vi "Kinect Track Demo.vi"() -> ()   [LabVIEW 2010]
uses:
  Kinect_API.lvlib
  labview-trunk/vi/clearpath_interface.lvlib
  <vilib>/Platform/TimedLoop/XDataNode/wakeup.ctl
  <vilib>/Platform/TimedLoop/XDataNode/XDNodeRunTimeDep.lvlib
  <vilib>/Platform/TimedLoop/XDataNode/nitl_modes.ctl
  <vilib>/Platform/TimedLoop/XDataNode/timing_clust.ctl
  <vilib>/Platform/TimedLoop/XDataNode/XDataNode.xnode
  cpp_lv.dll
panel:
  in  "Stop Husky":bool=TRUE
  in  "Tab Control":T1(tab)
  out "Depth":T2(plugin-control)
  out "Video":T2(plugin-control)
  in  "Wait For Next Image?":bool
  out "Depth Image Pixels (U16)":u16[][](array[numeric])
  out "Video Image Pixels (U32)":u32[][](array[numeric])
  out "Image Is New? (Video)":bool
  out "Image Is New? (Depth)":bool
  in  "Remove Zeros?":bool=TRUE
  in  "Focal Length in Pixels":dbl=285.63
  out "Iteration Delay":u32
  out "Mean Delay (N=100)":dbl
  out "Approx. FPS":dbl
  in  "Wall Buffer":dbl=0.7 min=0.0 step=0.1
  in  "FollowModeOn":bool=TRUE
  out "Linear Velocity":dbl(knob) scale=-1.0..1.0
  out "Angular Velocity":dbl(knob) scale=2.0..-2.0
  in  "Serial Port":refnum<visa-resource-name>="COM1"
  in  "Linear Speed":dbl=0.3 min=0.0 max=1.0 step=0.1
  in  "Angular Speed":dbl=0.2 min=0.0 max=2.0 step=0.1
  in  "Window Size":dbl=0.5 min=0.0 step=0.1
  in  "stop":bool
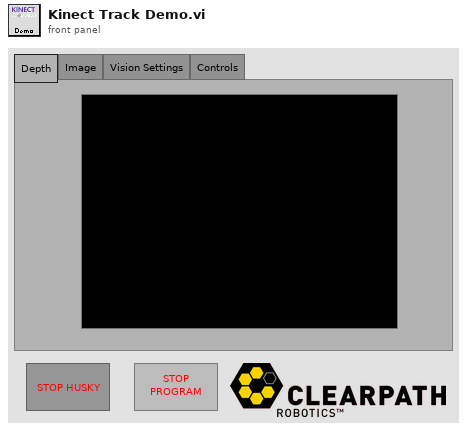
[diagram p1: front panel]
types:
  T1 = enum32{"Depth", "Image", "Vision Settings", "Controls"}
  T2 = typedef "IMAQ Image.ctl" = refnum<image>
  T3 = cluster{"Xmit Queue":refnum<queue>, "Data Queue":refnum<queue>, "VISA resource name out":refnum<visa-resource-name>, "error out":errorcluster, "Message Data Cluster":cluster{"\nChar Idx":u8, "Num. Char Rem":u8, "Write Index":u8, "Read Index":u8, "Message Data Buffer":u8[][]}}
  T4 = typedef "XDNodeRunTimeDep.lvlib/timing_clust.ctl" = cluster{"Expected End [f-1]":u64, "Actual End [f-1]":u64, "Finished Late? [f-1]":bool, "Expected End [i-1]":u64, "Actual End [i-1]":u64, "Finished Late? [i-1]":bool, "Expected Start [i]":u64, "Actual Start [i]":u64, "Expected Start [f]":u64, "Actual Start [f]":u64, "Source Name":string, "Structure Name":string, "Period":i64, "Deadline":i64, "Offset":i64, "Start":i64, "Priority":i32, "Timeout":i32, "Mode":T5, "Wakeup Reason":T6, "Error":errorcluster, "Source Type":string, "Secondary Source Type":string, "Global End Time":u64, "Global Start Time":u64, "Frame Duration":u64, "Iteration Duration":u64, "Assigned CPU":i32, "I/O Scan Engine Mode":u32}
  T5 = typedef "XDNodeRunTimeDep.lvlib/nitl_modes.ctl" = enum32{"No Change", "Process missed periods, maintain original phase", "Discard missed periods, maintain original phase", "Process missed periods, ignore original phase", "Discard missed periods, ignore original phase"}
  T6 = typedef "XDNodeRunTimeDep.lvlib/wakeup.ctl" = enum32{"Normal", "Aborted", "Asynchronous wakeup", "Timing source error", "Timed loop error", "Timeout"}
  T7 = cluster{"queue out":refnum<queue>, "queue out":refnum<queue>}
  T8 = cluster{"new reference":refnum<k24>, "DepthStream":refnum<k24>, "VideoStream":refnum<k24>, "Event Callback":refnum<k27>, "Event Callback":refnum<k27>}
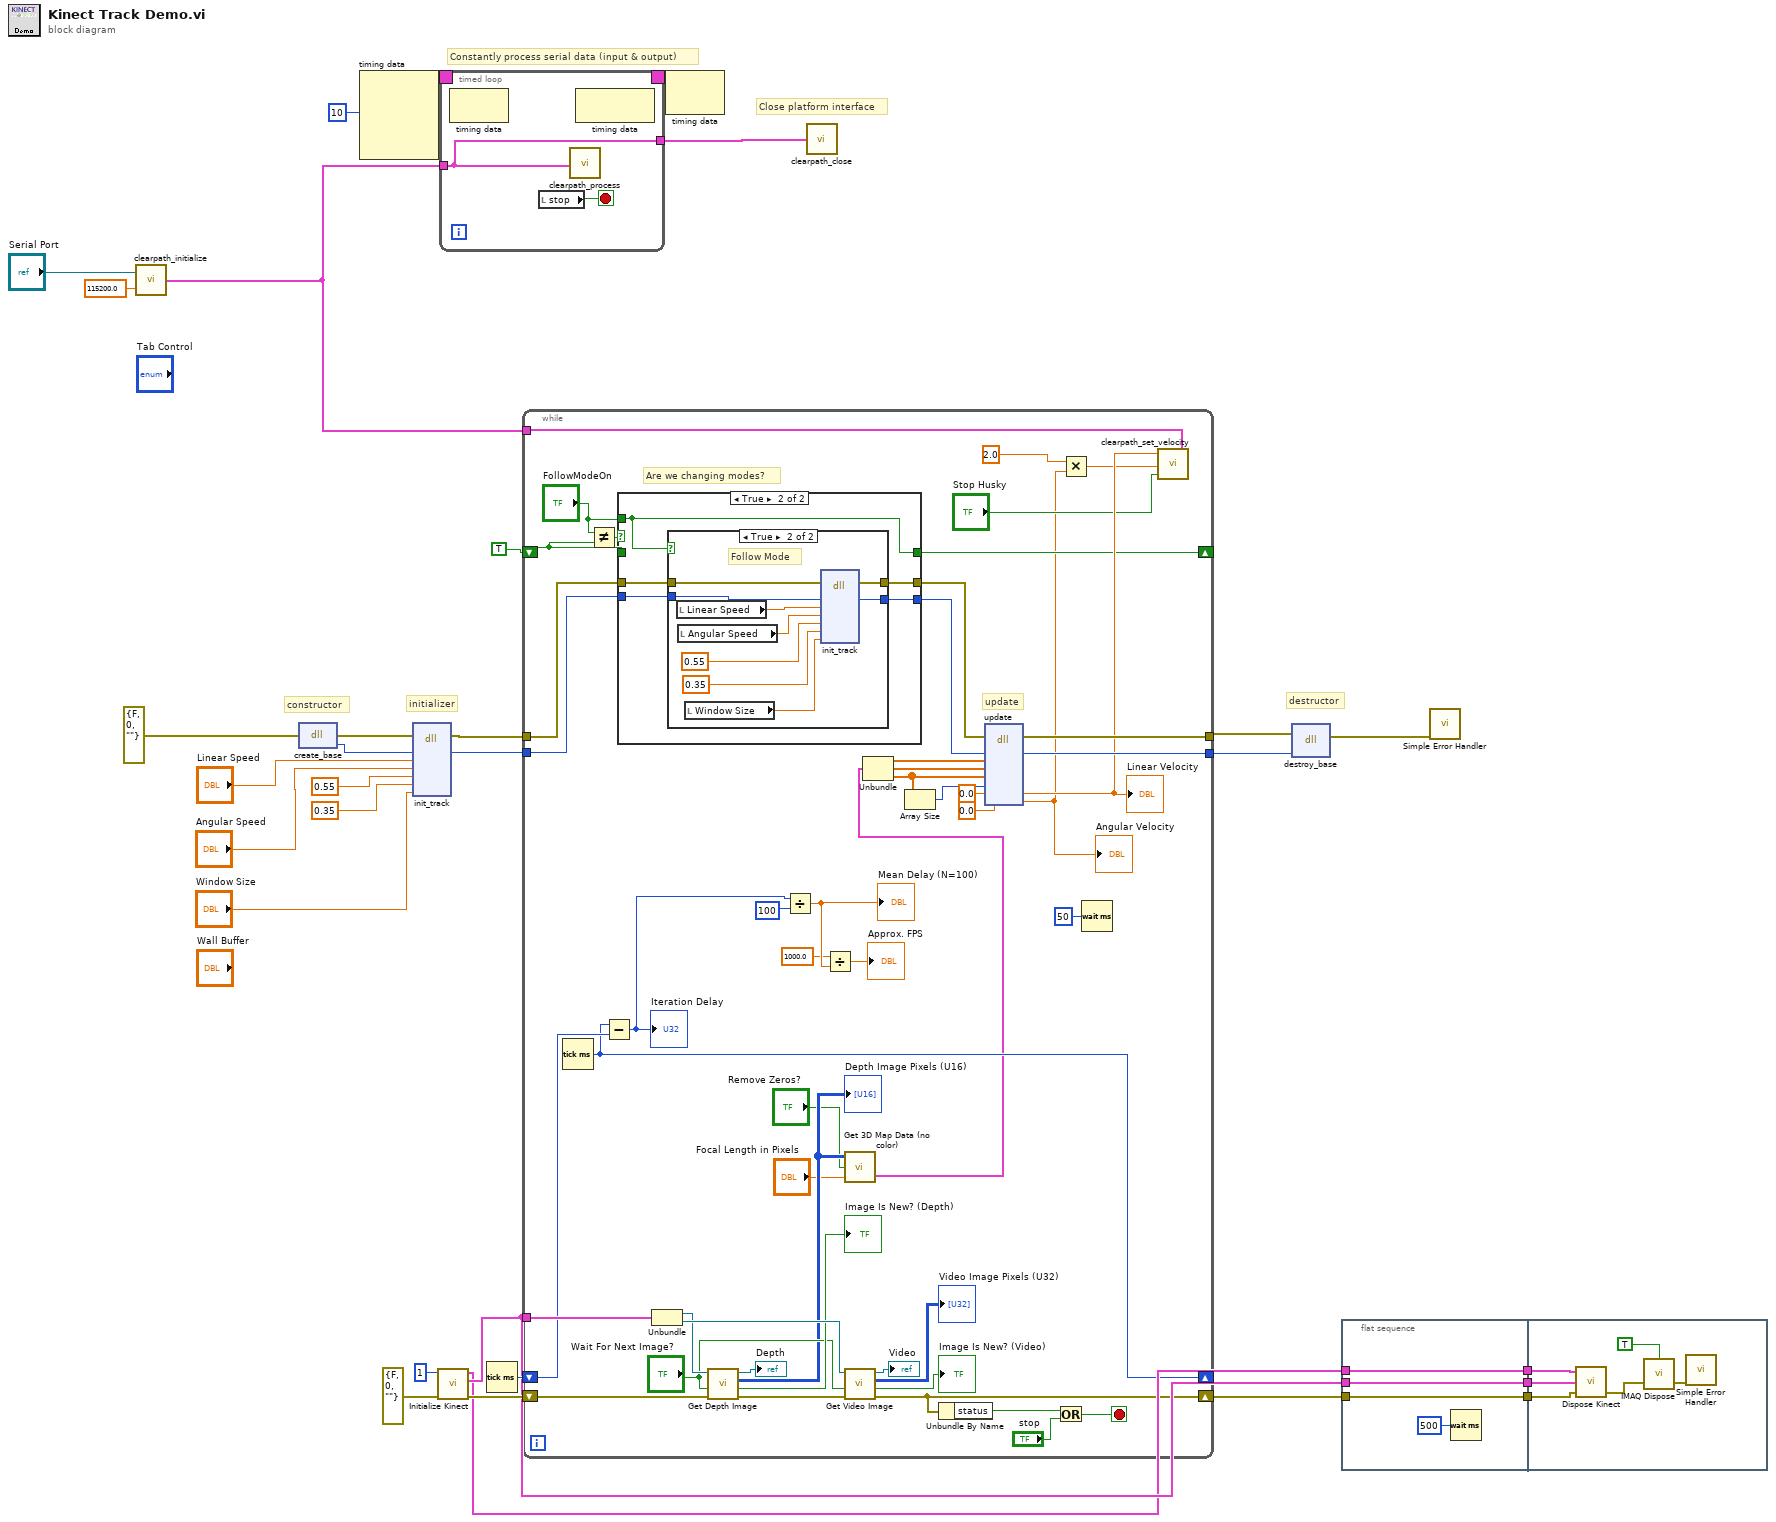
[diagram p0: block diagram]
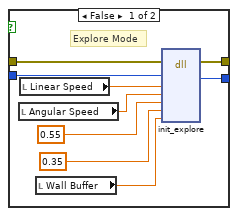
[diagram p3: hidden frame]
diagram:
  # "destructor"
  # "initializer"
  # "constructor"
  # "Constantly process serial data (input & output)"
  # "Close platform interface"
  n1 = call "clearpath_initialize.vi"("Baud rate"=115200.0, "VISA resource name"="Serial Port") -> ("ClearpathComm"=w31:T3)
  n2 = dll-call lib="C:/Users/clearpath/Desktop/Kinect Demo/cpp_lv.dll" fn="create_base"(error in=errorcluster {"status"=FALSE, "code"=0, "source"=""} ("error in (no error)")) -> (error out=w9:errorcluster, "LV_ref"=w8:u32)  [unwired: 2 in, 1 out]
  n3 = node-c288(i64 10 ("Period")) -> (w15:T4)  [unwired: 3 in]
  n4 = dll-call lib="C:/Users/clearpath/Desktop/Kinect Demo/cpp_lv.dll" fn="init_track"(error in=w9, "LV_ref"=w8, "lin_speed"="Linear Speed", "ang_speed"="Angular Speed", "cam_height"=0.55, "cam_z_trans"=0.35, "window_size"="Window Size") -> (error out=w18:errorcluster, "LV_ref"=w17:u32)  [unwired: 8 in, 1 out]
  n5 = call "Initialize Kinect.vi"("error in (no error)"=errorcluster {"status"=FALSE, "code"=0, "source"=""}, "Buffer Size"=1) -> ("error out"=w27:errorcluster, "Queues Out"=w23:T7, "References"=w22:T8)  [unwired: 7 in]
  n6 = timed-loop {
    tunnel: w31 -> [w33]
    tunnel: [w33] -> w13
    timing: w15 -> [_]
    timing-out: [_] -> w14
    stop <- w32 stop-if-true
    n7 = node-c288() -> ()  [unwired: 1 in, 1 out]
    n8 = local read "stop"() -> (w32:bool)
    n9 = call "clearpath_process.vi"("ClearpathComm"=w33) -> ()
    n10 = node-c288() -> ()  [unwired: 1 in, 1 out]
  }
  n11 = Tick Count (ms)() -> (millisecond timer value=w24:u32)
  n12 = while {
    tunnel: w23 -> [w84]
    shift-right: [w72] -> w21
    shift-left: w27 -> [w74]
    shift-right: [w65] -> _
    shift-left: w24 -> [w66]
    tunnel: [w59] -> w20
    tunnel: [w58] -> w19
    tunnel: w18 -> [w44]
    tunnel: w17 -> [w43]
    tunnel: w31 -> [w52]
    shift-right: [w48] -> _
    shift-left: TRUE ("FollowModeOn") -> [w47]
    stop <- w77 stop-if-true
    # "Are we changing modes?"
    # "update"
    n13 = Tick Count (ms)() -> (millisecond timer value=w65:u32)
    n14 = Not Equal?(x="FollowModeOn", y=w47) -> (x != y?=w36:bool)
    n15 = Subtract(x=w65, y=w66) -> (x-y=w39:u32)
    "Iteration Delay" <- w39
    n16 = case shown="True" w36 {
      tunnel: [w87 w92] -> w48
      tunnel: "FollowModeOn" -> [_ w92]
      tunnel: w47 -> [w87 _]
      tunnel: [w86 w91] -> w46
      tunnel: [w85 w90] -> w45
      tunnel: w44 -> [w86 w89]
      tunnel: w43 -> [w85 w88]
      frame False {
      }
      frame True {
        n17 = case shown="True" w92 {
          tunnel: [w101 w110] -> w91
          tunnel: [w100 w109] -> w90
          tunnel: w89 -> [w99 w108]
          tunnel: w88 -> [w98 w107]
          frame False {
            # "Explore Mode"
            n18 = local read "Angular Speed"() -> (w93:dbl)
            n19 = local read "Linear Speed"() -> (w97:dbl)
            n20 = local read "Wall Buffer"() -> (w96:dbl)
            n21 = dll-call lib="C:/Users/clearpath/Desktop/Kinect Demo/cpp_lv.dll" fn="init_explore"(error in=w99, "LV_ref"=w98, "lin_speed"=w97, "ang_speed"=w93, "cam_height"=0.55, "cam_z_trans"=0.35 ("cam_height"), "wall_buffer"=w96) -> (error out=w101:errorcluster, "LV_ref"=w100:u32)  [unwired: 8 in, 1 out]
          }
          frame True {
            # "Follow Mode"
            n22 = local read "Linear Speed"() -> (w106:dbl)
            n23 = local read "Angular Speed"() -> (w105:dbl)
            n24 = local read "Window Size"() -> (w104:dbl)
            n25 = dll-call lib="C:/Users/clearpath/Desktop/Kinect Demo/cpp_lv.dll" fn="init_track"(error in=w108, "LV_ref"=w107, "lin_speed"=w106, "ang_speed"=w105, "cam_height"=0.55, "cam_z_trans"=0.35, "window_size"=w104) -> (error out=w110:errorcluster, "LV_ref"=w109:u32)  [unwired: 8 in, 1 out]
          }
        }
      }
    }
    n26 = Unbundle(w84) -> ("queue out"=w71:refnum<queue>, "queue out"=w82:refnum<queue>)
    n27 = call "Get Depth Image.vi"("error in (no error)"=w74, "Wait For Next Image?"="Wait For Next Image?", "queue in"=w71) -> ("error out"=w73:errorcluster, "Image Is New?"=→"Image Is New? (Depth)":bool, "Depth Image Pixels (U16)"=w69:u16[][], "Depth Image"=→"Depth":T2)  [unwired: 5 in]
    "Depth Image Pixels (U16)" <- w69
    n28 = Divide(x=w39, y=u32 100) -> (x/y=w63:dbl)
    "Mean Delay (N=100)" <- w63
    n29 = Divide(x=1000.0, y=w63) -> (x/y=→"Approx. FPS":dbl)
    n30 = call "Get 3D Map Data (no color).vi"("Focal Length in Pixels"="Focal Length in Pixels", "Remove Zeros?"="Remove Zeros?", "Depth Image Pixels (U16) In"=w69) -> ("3D Information Cluster (X,Y,Z)"=w57:cluster{dbl[], dbl[], dbl[]})  [unwired: 1 out]
    n31 = call "Get Video Image.vi"("error in (no error)"=w73, "Wait For Next Image?"="Wait For Next Image?", "queue in"=w82) -> ("error out"=w72:errorcluster, "Image Is New?"=→"Image Is New? (Video)":bool, "Video Image Pixels (U32)"=→"Video Image Pixels (U32)":u32[][], "Video Image"=→"Video":T2)  [unwired: 5 in]
    n32 = Unbundle(w57) -> (w56:dbl[], w55:dbl[], w54:dbl[])
    n33 = Array Size(array=w54) -> (size(s)=w53:i32)
    n34 = Unbundle By Name(w72) -> ("status"=w79:bool)
    n35 = dll-call lib="C:/Users/clearpath/Desktop/Kinect Demo/cpp_lv.dll" fn="update"(error in=w46, "LV_ref"=w45, "px"=w56, "py"=w55, "pz"=w54, "len"=w53, "return_lin_vel"=0.0, "return_ang_vel"=0.0) -> (error out=w58:errorcluster, "LV_ref"=w59:u32, "return_lin_vel"=w51:dbl, "return_ang_vel"=w41:dbl)  [unwired: 7 in, 1 out]
    "Linear Velocity" <- w51
    "Angular Velocity" <- w41
    n36 = Or(x=w79, y="stop") -> (x .or. y?=w77:bool)
    n37 = Multiply(x=2.0 ("y"), y=w41) -> (x*y=w50:dbl)
    n38 = Wait (ms)(milliseconds to wait=u32 50) -> ()  [unwired: 1 out]
    n39 = call "clearpath_set_velocity.vi"("ClearpathComm"=w52, "Zero Speeds"="Stop Husky", "Rotational Speed"=w50, "Translational Speed"=w51) -> ()
  }
  n40 = node-c288(w14) -> ()  [unwired: 1 out]
  n41 = call "clearpath_close.vi"("ClearpathComm"=w13) -> ()
  n42 = dll-call lib="C:/Users/clearpath/Desktop/Kinect Demo/cpp_lv.dll" fn="destroy_base"(error in=w19, "LV_ref"=w20) -> (error out=w1:errorcluster)  [unwired: 4 in, 1 out]
  n43 = flat-sequence {
    tunnel: [w114] -> w30
    tunnel: w23 -> [w114]
    tunnel: [w113] -> w29
    tunnel: w22 -> [w113]
    tunnel: [w112] -> w28
    tunnel: w21 -> [w112]
    tunnel: w30 -> [w117]
    tunnel: w29 -> [w116]
    tunnel: w28 -> [w115]
    frame #0 {
      n44 = Wait (ms)(milliseconds to wait=u32 500) -> ()  [unwired: 1 out]
    }
    frame #1 {
      n45 = call "Dispose Kinect.vi"("error in (no error)"=w115, "Queues In"=w117, "References"=w116) -> ("error out"=w119:errorcluster)  [unwired: 2 in]
      n46 = call "IMAQ Dispose"("All Images? (No)"=TRUE, "error in (no error)"=w119) -> ("error out"=w120:errorcluster)  [unwired: 4 in]
      n47 = call <vilib>:"Simple Error Handler.vi"("error in (no error)"=w120) -> ()  [unwired: 4 in, 5 out]
    }
  }
  n48 = call <vilib>:"Simple Error Handler.vi"("error in (no error)"=w1) -> ()  [unwired: 4 in, 5 out]
